vi "UDP数据接收循环.vi"(7 "停止采集":bool, 8 "错误输入（无错误）":errorcluster, 10 "结束位队列":refnum<queue>, 11 "队列输入":refnum<queue>) -> (2 "状态显示":string)   [LabVIEW 2020]
panel:
  out "解析后数据":i32[][](array[numeric])
  in  "数据采集卡地址":string
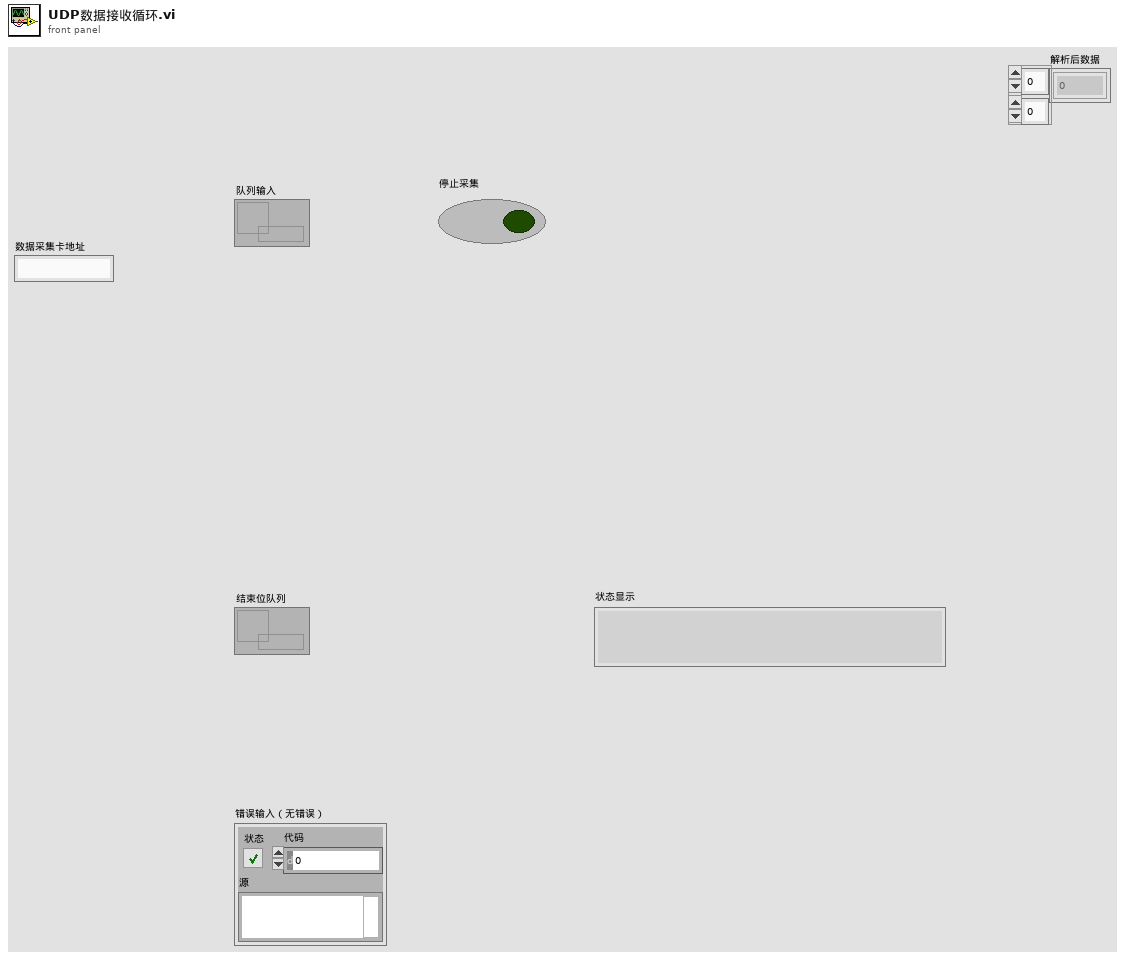
[diagram p1: front panel]
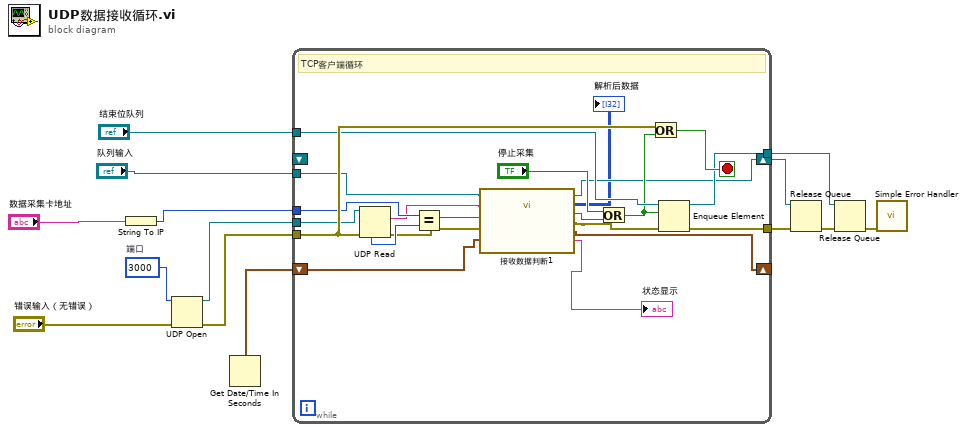
[diagram p0: block diagram]
diagram:
  w1 = u16 3000  # 端口
  n1 = String To IP(1:"数据采集卡地址") -> (0:w12:u32)
  n2 = UDP Open(8:"错误输入（无错误）", 11:w1) -> (port=w3:refnum<k16>, 0:w4:errorcluster)  [unwired: 3 in, 1 out]
  n3 = Get Date/Time In Seconds() -> (seconds since 1Jan1904=w13:timestamp)
  n4 = while {
    tunnel: w4 -> [w34]
    tunnel: w3 -> [w33]
    tunnel: "结束位队列" -> [w32]
    tunnel: [w31] -> w7
    tunnel: "队列输入" -> [w25]
    shift-right: [w20] -> w9
    shift-left: _ -> [_]
    tunnel: w12 -> [w29]
    shift-right: [w17] -> _
    shift-left: w13 -> [w21]
    tunnel: [w27] -> w14
    stop <- w35 stop-if-true
    # "TCP客户端循环"
    n5 = UDP Read(connection ID=w33, 8:w34) -> (data out=w24:string, error out=w22:errorcluster, 6:w30:u32)  [unwired: 1 in, 3 out]
    n6 = Equal?(x=w29, y=w30) -> (x = y?=w23:bool)
    n7 = call "接收数据判断1.vi"("上次正确接收数据时间"=w21, "错误输入（无错误）"=w22, "IP地址比较位"=w23, "data out"=w24, "队列输入"=w25) -> ("错误输出"=w18:errorcluster, "结束标志位"=w19:bool, "解析后数据"=→"解析后数据":i32[][], "队列输出"=w20:refnum<queue>, "正确接收数据时间"=w17:timestamp, "状态显示"=→"状态显示":string)  [unwired: 1 in]
    n8 = Or(x="停止采集", y=w19) -> (x .or. y?=w26:bool)
    n9 = Or(x=w34, y=w26) -> (x .or. y?=w35:bool)
    n10 = Enqueue Element(queue=w32, element=w26, error in (no error)=w18) -> (queue out=w31:refnum<queue>, error out=w27:errorcluster)  [unwired: 1 in, 1 out]
  }
  n11 = Release Queue(queue=w9, error in (no error)=w14) -> (error out=w5:errorcluster)  [unwired: 1 in, 2 out]
  n12 = Release Queue(queue=w7, error in (no error)=w5) -> (error out=w6:errorcluster)  [unwired: 1 in, 2 out]
  n13 = call <vilib>:"Simple Error Handler.vi"("error in (no error)"=w6) -> ()  [unwired: 4 in, 5 out]
